vi "SRflipFlop.vi"(9 "R":bool, 10 "Clk":bool, 11 "S":bool) -> (2 "Q":bool, 3 "/Q\\":bool)   [LabVIEW 2012]
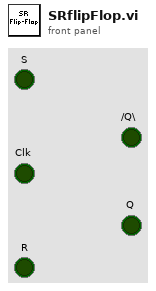
[diagram p1: front panel]
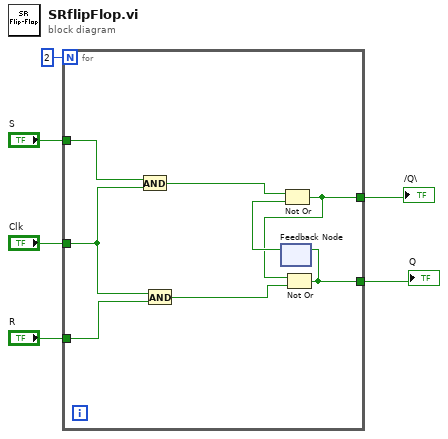
[diagram p0: block diagram]
diagram:
  n1 = for {
    N: 2 -> [_]
    tunnel: "S" -> [w11]
    tunnel: "Clk" -> [w10]
    tunnel: "R" -> [w9]
    tunnel: [w8] -> w3
    tunnel: [w7] -> w2
    n2 = And(x=w11, y=w10) -> (x .and. y?=w13:bool)
    n3 = And(x=w10, y=w9) -> (x .and. y?=w12:bool)
    n4 = feedback #1() -> (w14:bool)  [unwired: 1 in]
    n5 = Not Or(1:w14, 2:w13) -> (0:w7:bool)
    n6 = Not Or(1:w12, 2:w7) -> (0:w8:bool)
    n7 = feedback-in #1(w8) -> ()
  }
  "Q" <- w3
  "/Q\\" <- w2
